vi "Lock Controls.vi"(8 "error in (no error)":errorcluster, 10 "Lock Controls?":bool, 11 "PicoScope 3000a in":refnum<class "PicoScope 3000a.lvclass">) -> (0 "error out":errorcluster, 3 "PicoScope 3000a out":refnum<class "PicoScope 3000a.lvclass">)   [LabVIEW 2018, in "PicoScope 3000a.lvlib" / "PicoScope 3000a.lvclass"]
doc: "This override method is used to lock/unlock user access to the oscilloscope front panel controls."
uses:
  PicoScope 3000a.lvclass
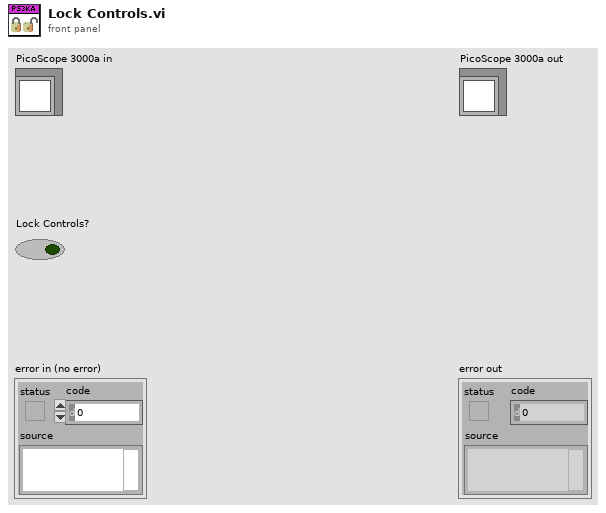
[diagram p1: front panel]
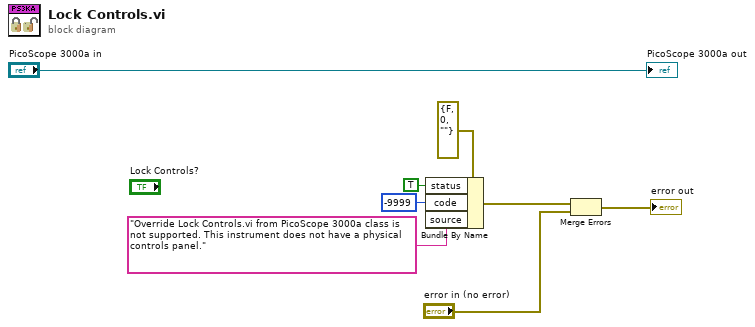
[diagram p0: block diagram]
diagram:
  n1 = Bundle By Name(cluster=errorcluster {"status"=FALSE, "code"=0, "source"=""} ("error constant"), "status"=TRUE, "code"=-9999, "source"="Override Lock Controls.vi from PicoScope 3000a class is not supported. This instrument does not have a physical controls panel.") -> (w3:errorcluster)
  n2 = Merge Errors(w3, "error in (no error)") -> (→"error out":errorcluster)
  "PicoScope 3000a out" <- "PicoScope 3000a in"
